vi "Init.vi"(8 "error in (no error)":errorcluster, 9 "ICameraTesting":refnum<class "ICameraTesting.lvclass">, 10 "CameraInfo":T1, 11 "ICameraTestingProxy in":refnum<class "ICameraTestingProxy.lvclass">) -> (0 "error out":errorcluster, 3 "ICameraTestingProxy out":refnum<class "ICameraTestingProxy.lvclass">)   [LabVIEW 2020, in "ICameraTestingProxy.lvlib" / "ICameraTestingProxy.lvclass"]
uses:
  ICameraTestingProxy.lvclass
  Camera/ICamera/ICamera/ICamera.lvclass
  CameraTestingApp/ICameraTesting/ICameraTesting/ICameraTesting.lvclass
  CameraTestingApp/ICameraTesting/TypeDef/CameraInfo.ctl
  CameraTestingApp/ICameraTesting/TypeDef/ICameraTesting_typedef.lvlib
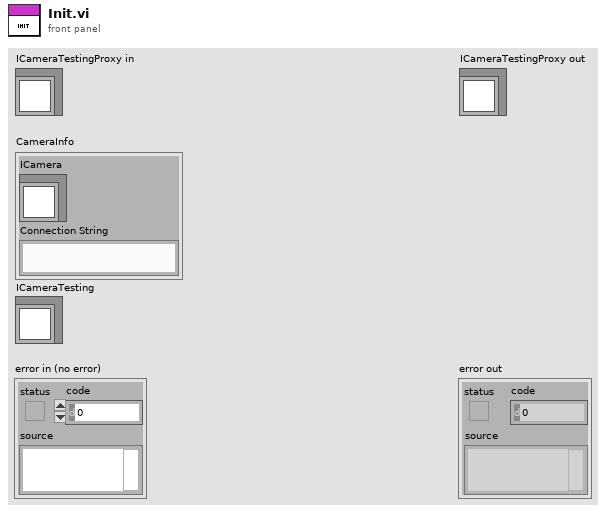
[diagram p1: front panel]
types:
  T1 = typedef "ICameraTesting_typedef.lvlib/CameraInfo.ctl" = cluster{"ICamera ":refnum<class "ICamera.lvclass">, "Connection String":string}
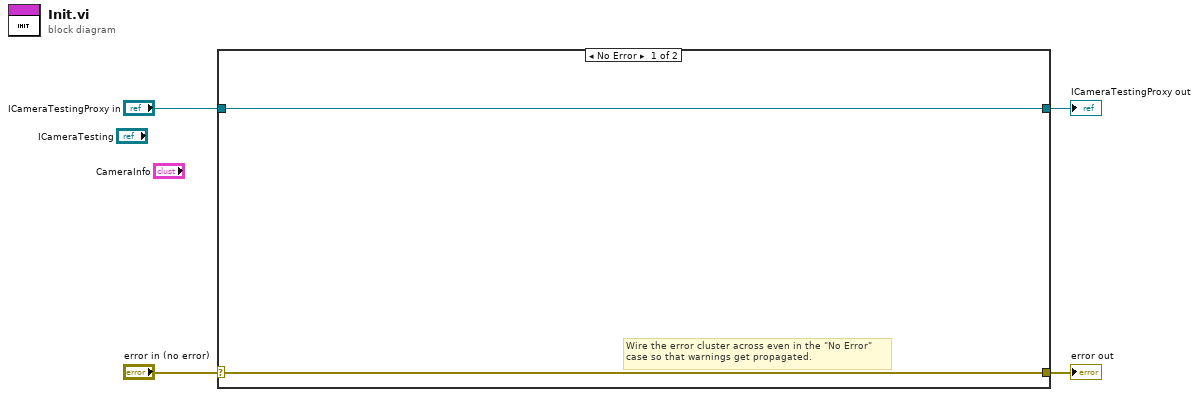
[diagram p0: block diagram]
diagram:
  n1 = case shown="No Error" "error in (no error)" {
    selector: "error in (no error)" -> [w5 w8]
    tunnel: [w5 w8] -> w3
    tunnel: [w6 w7] -> w1
    tunnel: "ICameraTestingProxy in" -> [w6 w7]
    frame No Error {
      # "Wire the error cluster across even in the \"No Error\"\ncase so that warnings get propagated."
    }
    frame Error {
    }
  }
  "error out" <- w3
  "ICameraTestingProxy out" <- w1
